vi "SVT Build Result Table (N Ch).vi"(0 "octave spectra":T5(array[cluster]) {"band power" format="%.2f"; "nominal frequencies [Hz]" format="%.2f"}, 5 "precision (1)":i16=1 min=0, 9 "octave info":T1[](array[typedef]) {"engineering units" items=["custom..."=0, "V"=1, "A"=21, "C"=30, "pC"=31, "s"=32, "-"=29, "Pa"=2, "N"=20, "g"=3, "m/s^2"=4, "m/s"=5, "m"=6, "mm/s"=12, "mm"=13, "micron/s"=14, "micron"=15, "in/s^2"=7, "in/s"=8, "in"=9, "mil/s"=10, "mil"=11, "rad/s^2"=16, "rad/s"=17, "rad"=18, "deg/s^2"=26, "deg/s"=27, "deg"=28, "RPM"=22, "cycle/s^2"=23, "Hz"=24, "cycle"=25, "strain"=19]; "dB reference" format="%.2e"; "weighting filter" items=["Linear", "A-weighting", "B-weighting", "C-weighting", "ITU-R 468-4", "Dolby", "CCITT", "C-message", "Wb", "Wc", "Wd", "We", "Wf", "Wh", "Wj", "Wk", "Wm", "AES17 20 kHz lowpass", "AES17 40 kHz lowpass", "AES17 20 kHz highpass", "AES17 40 kHz highpass"]}, 11 "error in (no error)":errorcluster, 12 "include units with values (T)":bool=TRUE) -> (4 "result table":string[][](table), 6 "column headers":string[](array[string]), 15 "error out":errorcluster)   [LabVIEW 2017, in "SoundVib_Octave.lvlib"]
doc: "Generates a table of the results of a fractional-octave analysis. The first column of the table contains the nominal frequencies in Hz. The second and subsequent columns contain the 1/n band power with the appropriate unit label. Wire data to the <B>octave spectrum</B> input to determine the polymorphic instance to use or manually select the instance."
uses:
  <vilib>/addons/Sound and Vibration/svt_Octave/SoundVib_Octave.lvlib
  <vilib>/addons/_NISVFA/_Shared subVIs/Controls/svc_Octave Info.ctl
  <vilib>/addons/_NISVFA/_Shared subVIs/Controls/svc_Octave Standard.ctl
  <vilib>/addons/_NISVFA/_Shared subVIs/Controls/svc_Weighting Filter Text Ring.ctl
  <vilib>/addons/_NISVFA/_Shared subVIs/Controls/svc_Engineering Units Text Ring.ctl
  <vilib>/addons/_NISVFA/_Shared subVIs/Common/svc_Sort XY Results.vi
  <vilib>/addons/Sound and Vibration/svt_Octave_2014 standard/SoundVib_Octave_2014 standard.lvlib
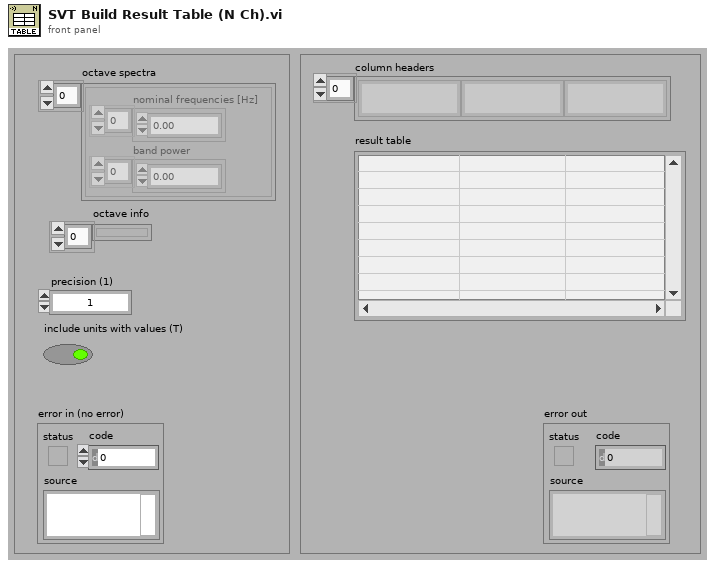
[diagram p1: front panel]
types:
  T1 = typedef "svc_Octave Info.ctl" = cluster{"standard":T2, "bandwidth":enum16{"1 octave", "1/3 octave", "1/6 octave", "1/12 octave", "1/24 octave"}, "low band":i32, "high band":i32, "weighting filter":T3, "dB reference":dbl, "dB On":bool, "unit label":string, "channel name":string, "description":string, "engineering units":T4, "custom label":string, "spectrum type":enum16{"power", "magnitude"}, "spectral density":bool, "filters settled":bool}
  T2 = typedef "svc_Octave Standard.ctl" = enum16{"ANSI S1.11", "IEC 61260"}
  T3 = typedef "svc_Weighting Filter Text Ring.ctl" = u16
  T4 = typedef "svc_Engineering Units Text Ring.ctl" = u16
  T5 = cluster{"nominal frequencies [Hz]":dbl[], "band power":dbl[]}[]
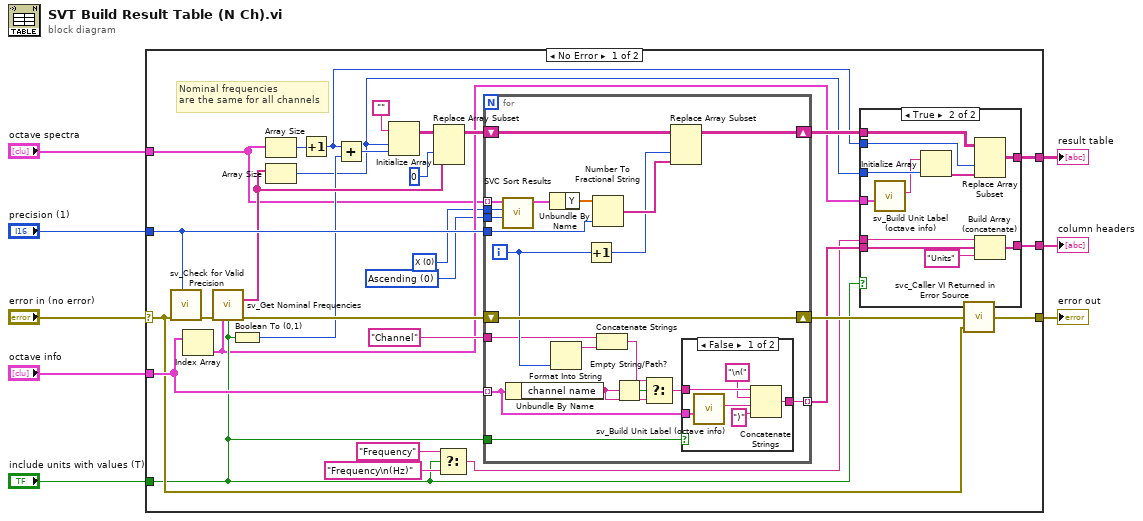
[diagram p0: block diagram]
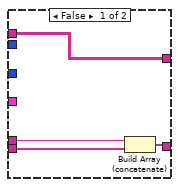
[diagram p2: hidden frame]
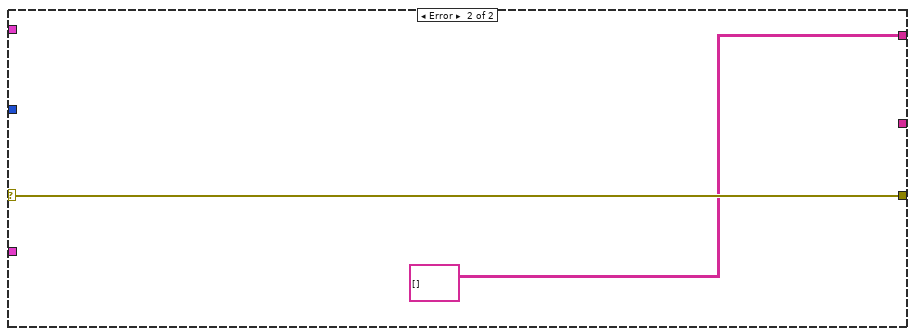
[diagram p4: hidden frame]
diagram:
  n1 = case shown="No Error" "error in (no error)" {
    selector: "error in (no error)" -> [w25 w83]
    tunnel: "octave info" -> [w28 _]
    tunnel: "precision (1)" -> [w30 _]
    tunnel: "octave spectra" -> [w11 _]
    tunnel: [w32 string[][] []] -> w5
    tunnel: [w31 w83] -> w4
    tunnel: "include units with values (T)" -> [w16 _]
    tunnel: [w23 _] -> w1
    frame No Error {
      w9 = u16 0 items=["Ascending", "Descending"] ("sort order")
      w10 = u16 0 items=["X", "Y"] ("sort by")
      # "Nominal frequencies \nare the same for all channels"
      n2 = call <vilib>:"sv_Check for Valid Precision.vi"("precision (1)"=w30, "error in (no error)"=w25) -> ("error out"=w29:errorcluster)  [unwired: 9 in]
      n3 = Index Array(array=w28) -> (element=w12:T1)  [unwired: 1 in]
      n4 = call <vilib>:"sv_Get Nominal Frequencies.vi"("error in (no error)"=w29, "octave info"=w12, "include units (T)"=w16) -> ("nominal frequencies (string)"=w22:string[], "error out"=w26:errorcluster)  [unwired: 10 in, 1 out]
      n5 = Boolean To (0,1)(Boolean=w16) -> (0, 1=w15:i16)
      n6 = Array Size(array=w11) -> (size(s)=w35:i32)
      n7 = Array Size(array=w22) -> (size(s)=w13:i32)
      n8 = Increment(x=w35) -> (x+1=w14:i32)
      n9 = Add(x=w14, y=w15) -> (x+y=w34:i32)
      n10 = Initialize Array("", w13, w34) -> (w38:string[][])
      n11 = Replace Array Subset(array=w38, new element=w22, index (col)=0 ("Disabled Index (col)")) -> (w37:string[][])  [unwired: 1 in]
      n12 = Select(t="Frequency", s=w16, f="Frequency\n(Hz)") -> (s? t:f=w18:string)
      n13 = for {
        tunnel: w11 -> [w57] mode=indexing
        tunnel: w28 -> [w58] mode=indexing
        tunnel: w30 -> [w67]
        shift-right: [w73] -> w33
        shift-left: w37 -> [w74]
        shift-right: [w65] -> w27
        shift-left: w26 -> [w65]
        tunnel: [w68] -> w24 mode=indexing
        tunnel: w16 -> [w60]
        tunnel: "Channel" -> [w59]
        tunnel: w10 -> [w55]
        tunnel: w9 -> [w54]
        i -> [w62]
        n14 = call-poly <vilib>:"SVC Sort Results.vi"("sort order"=w54, "sort by"=w55, "XY in"=w57) -> ("sorted XY"=w56:cluster{"X":dbl[], "Y":dbl[]})  [unwired: 7 in, 1 out]
        n15 = Unbundle By Name(w58) -> ("channel name"=w70:string)
        n16 = Unbundle By Name(w56) -> ("Y"=w64:dbl[])
        n17 = Format Into String(w62) -> (resulting string=w71:string)  [unwired: 3 in, 1 out]
        n18 = Increment(x=w62) -> (x+1=w63:i32)
        n19 = Number To Fractional String(number=w64, precision (6)=w67) -> (F-format string=w66:string[])  [unwired: 2 in]
        n20 = Concatenate Strings(w59, w71) -> (w61:string)
        n21 = Empty String/Path?(string/path=w70) -> (empty?=w72:bool)
        n22 = Select(t=w61, s=w72, f=w70) -> (s? t:f=w69:string)
        n23 = Replace Array Subset(array=w74, new element=w66, index (col)=w63) -> (w73:string[][])  [unwired: 1 in]
        n24 = case shown="False" w60 {
          tunnel: w69 -> [w80 w81]
          tunnel: [w79 w81] -> w68
          tunnel: w58 -> [w75 _]
          frame False {
            n25 = call <vilib>:"sv_Build Unit Label (octave info).vi"("octave info"=w75) -> ("unit label"=w76:string)  [unwired: 8 in, 2 out]
            n26 = Concatenate Strings(w80, "\n(" ("string"), w76, ")" ("string")) -> (w79:string)
          }
          frame True {
          }
        }
      }
      n27 = case shown="True" w16 {
        tunnel: w33 -> [w39 w53]
        tunnel: [w39 w52] -> w32
        tunnel: w24 -> [w42 w51]
        tunnel: [w41 w49] -> w23
        tunnel: w13 -> [_ w48]
        tunnel: w18 -> [w40 w46]
        tunnel: w14 -> [_ w45]
        tunnel: w12 -> [_ w44]
        frame False {
          n28 = Build Array (concatenate)(w40, w42) -> (w41:string[])
        }
        frame True {
          n29 = call <vilib>:"sv_Build Unit Label (octave info).vi"("octave info"=w44) -> ("unit label"=w43:string)  [unwired: 8 in, 2 out]
          n30 = Initialize Array(w43, w48) -> (w47:string[])
          n31 = Replace Array Subset(array=w53, new element=w47, index (col)=w45) -> (w52:string[][])  [unwired: 1 in]
          n32 = Build Array (concatenate)(w46, w51, "Units") -> (w49:string[])
        }
      }
      n33 = call <vilib>:"svc_Caller VI Returned in Error Source.vi"("warning input to caller"=w25, "error in (no error)"=w27) -> ("error out"=w31:errorcluster)  [unwired: 3 in]
    }
    frame Error {
    }
  }
  "result table" <- w5
  "error out" <- w4
  "column headers" <- w1
